vi "Time to wait before Triggering.vi"() -> ()   [LabVIEW 2022 SP3]
uses:
  Globals/Meas_global.vi
  Analysis/7 Hole Probe pressures to UVW/7HP_Global.vi
panel:
  out "ms to wait":i32
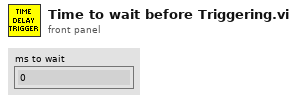
[diagram p1: front panel]
types:
  T1 = typedef "Device ID port info.ctl" = cluster{"Ch No":i16[], "Req Sampling Rate":dbl[], "Port":string, "Index":i32[]}
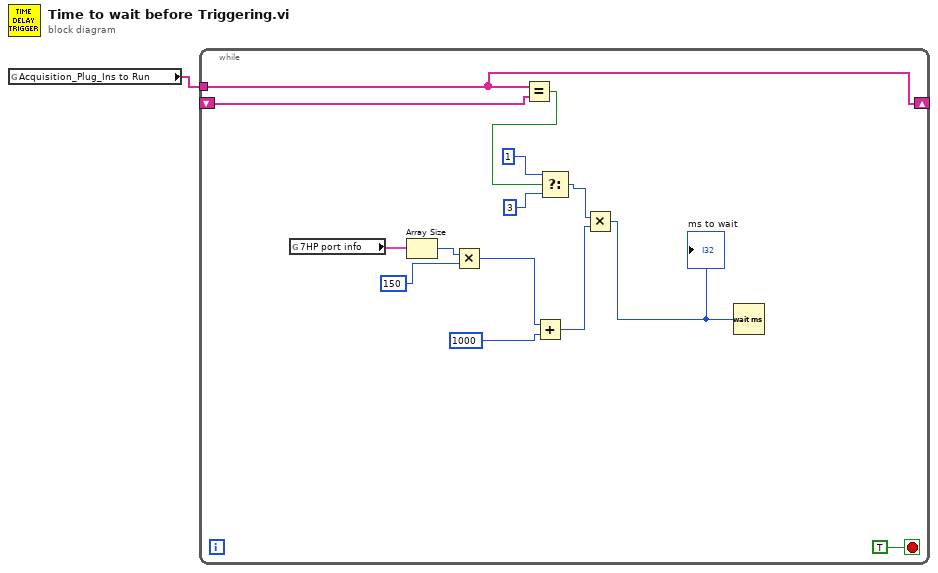
[diagram p0: block diagram]
diagram:
  n1 = global read "Meas_global.vi" "Acquisition_Plug_Ins to Run"() -> (w1:string[])
  n2 = while {
    shift-right: [w14] -> _
    shift-left: _ -> [w15]
    tunnel: w1 -> [w14]
    stop <- TRUE stop-if-true
    n3 = global read "7HP_Global.vi" "7HP port info"() -> (w12:T1[])
    n4 = Array Size(array=w12) -> (size(s)=w13:i32)
    n5 = Multiply(x=w13, y=150) -> (x*y=w9:i32)
    n6 = Equal?(x=w14, y=w15) -> (x = y?=w5:bool)
    n7 = Add(x=w9, y=1000 ("milliseconds to wait")) -> (x+y=w7:i32)
    n8 = Select(t=1, s=w5, f=3) -> (s? t:f=w2:i32)
    n9 = Multiply(x=w2, y=w7) -> (x*y=w6:i32)
    "ms to wait" <- w6
    n10 = Wait (ms)(milliseconds to wait=w6) -> ()  [unwired: 1 out]
  }
